vi "case_safe.vi"(6 "message cluster":T2, 7 "Main VI reference":refnum<vi>, 8 "error in (no error)":errorcluster, 9 "queue in":refnum<queue>, 10 "config refnum in":T1) -> (0 "error out":errorcluster, 2 "config refnum out":T1)   [LabVIEW 2020]
uses:
  controls/message cluster.ctl
  <vilib>/Utility/config.llb/Config Data RefNum.ctl
  23c514c1-82b2-402a-8425-70dfd9f23326.vi
  69df1d27-fced-4ab2-83d7-664410241a73.vi
  7ca75f6a-cbad-46dc-a29e-527fab8d5f55.vi
  ea2e0f2f-4b7c-4265-89be-48463285a396.vi
  <vilib>/Utility/config.llb/Write Key (String).vi
  <vilib>/Utility/config.llb/Write Key (Double).vi
  <vilib>/Utility/config.llb/NI_LVConfig.lvlib
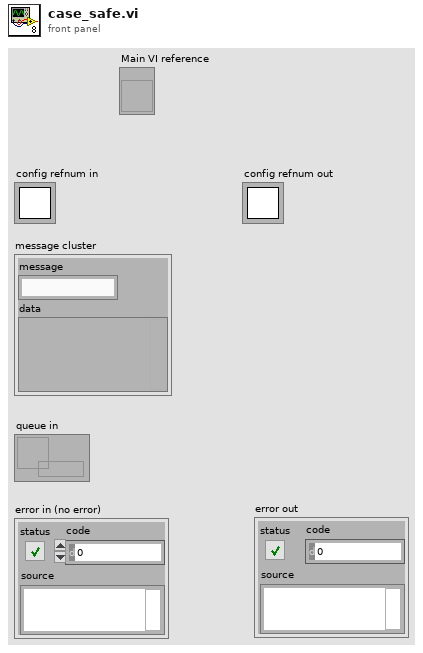
[diagram p1: front panel]
types:
  T1 = typedef "NI_LVConfig.lvlib/Config Data RefNum.ctl" = refnum<k1>
  T2 = typedef "message cluster.ctl" = cluster{"message":string, "data":variant}
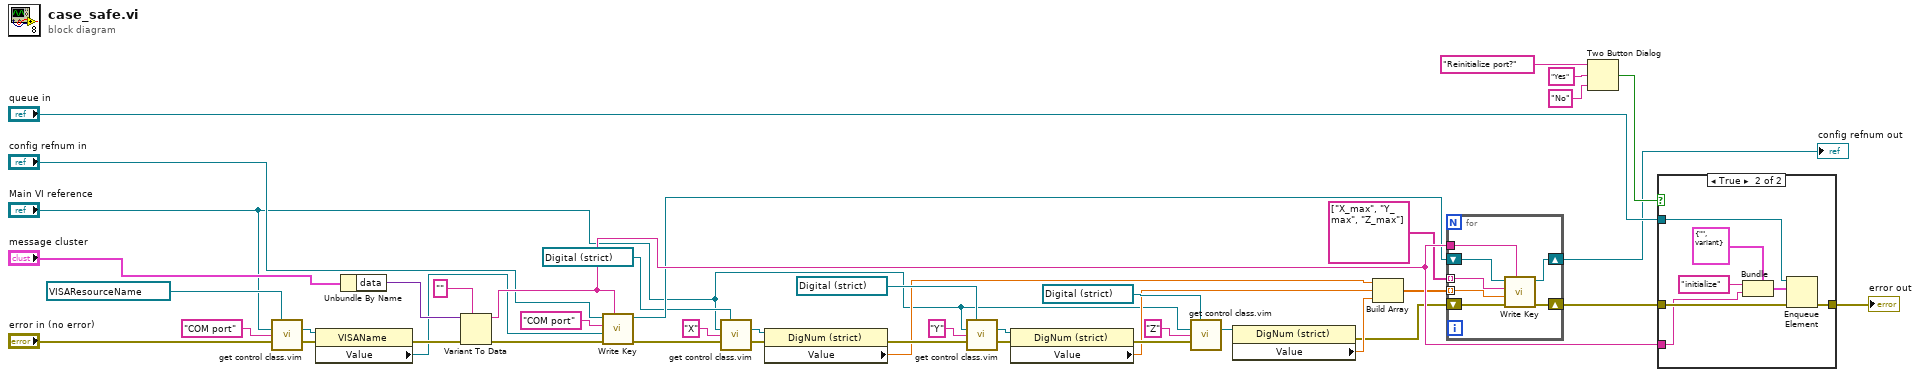
[diagram p0: block diagram]
diagram:
  n1 = call "get control class.vim"("Control class"=refnum<vi> refnum ("COM port"), "Main VI reference"="Main VI reference", "Label"="COM port", "error in (no error)"="error in (no error)") -> ("Control out"=w6:refnum<vi>, "error out"=w7:errorcluster)  [unwired: 10 in]
  n2 = property on="Property Node" class="VISAName"(reference=w6, error in=w7) -> (error out=w4:errorcluster, "Value"=w3:refnum<visa-resource-name>)  [unwired: 1 out]
  n3 = Unbundle By Name("message cluster") -> ("data"=w37:variant)
  n4 = Variant To Data(error in=w4, type="", Variant=w37) -> (data=w40:string, error out=w39:errorcluster)
  n5 = call-poly <vilib>:"Write Key.vi"("section"=w40, "error in (no error)"=w39, "value"=w3, "key"="COM port", "refnum"="config refnum in") -> ("error out"=w2:errorcluster, "refnum out"=w31:T1)  [unwired: 4 in, 1 out]
  n6 = call "get control class.vim"("Control class"=refnum<vi> refnum ("X"), "Main VI reference"="Main VI reference", "Label"="X", "error in (no error)"=w2) -> ("Control out"=w25:refnum<vi>, "error out"=w18:errorcluster)  [unwired: 10 in]
  n7 = property on="Property Node" class="DigNum (strict)"(reference=w25, error in=w18) -> (error out=w17:errorcluster, "Value"=w14:dbl)  [unwired: 1 out]
  n8 = call "get control class.vim"("Control class"=refnum<vi> refnum ("X"), "Main VI reference"="Main VI reference", "Label"="Y", "error in (no error)"=w17) -> ("Control out"=w22:refnum<vi>, "error out"=w16:errorcluster)  [unwired: 10 in]
  n9 = property on="Property Node" class="DigNum (strict)"(reference=w22, error in=w16) -> (error out=w15:errorcluster, "Value"=w13:dbl)  [unwired: 1 out]
  n10 = call "get control class.vim"("Control class"=refnum<vi> refnum ("X"), "Main VI reference"="Main VI reference", "Label"="Z", "error in (no error)"=w15) -> ("Control out"=w19:refnum<vi>)  [unwired: 10 in, 1 out]
  n11 = property on="Property Node" class="DigNum (strict)"(reference=w19) -> (error out=w1:errorcluster, "Value"=w12:dbl)  [unwired: 1 in, 1 out]
  n12 = Build Array(w14, w13, w12) -> (w11:dbl[])
  n13 = for {
    tunnel: w11 -> [w51] mode=indexing
    tunnel: string[] ["X_max", "Y_max", "Z_max"] -> [w50] mode=indexing
    shift-right: [w47] -> w34
    shift-left: w1 -> [w48]
    shift-right: [w46] -> w32
    shift-left: w31 -> [w49]
    tunnel: w40 -> [w45]
    n14 = call-poly <vilib>:"Write Key.vi"("section"=w45, "error in (no error)"=w48, "value"=w51, "key"=w50, "refnum"=w49) -> ("error out"=w47:errorcluster, "refnum out"=w46:T1)  [unwired: 4 in, 1 out]
  }
  "config refnum out" <- w32
  n15 = Two Button Dialog(message="Reinitialize port?", 1:"No" ("F button name (\"Cancel\")"), 2:"Yes" ("T button name (\"OK\")")) -> (T button?=w44:bool)
  n16 = case shown="True" w44 {
    tunnel: "queue in" -> [_ w59]
    tunnel: w34 -> [w52 w58]
    tunnel: [w52 w57] -> w35
    tunnel: w40 -> [_ w53]
    frame False {
    }
    frame True {
      n17 = Bundle(cluster=T2 {"message"="", "data"=variant}, "message"="initialize", "data"=w53) -> (w54:T2)
      n18 = Enqueue Element(queue=w59, element=w54, error in (no error)=w58) -> (error out=w57:errorcluster)  [unwired: 1 in, 2 out]
    }
  }
  "error out" <- w35
